vi "纳清pH电极校准.vi"() -> ()   [LabVIEW 2016, in "斯坦道多参数.lvlib"]
uses:
  <vilib>/Utility/miscctls.llb/LVPointTypeDef.ctl
  <vilib>/Analysis/NI_AALBase.lvlib
panel:
  out "第二点信号值":dbl
  out "第一点信号值":dbl
  out "报警信息":string
  out "通讯状态":string
  out "第二点校准值":dbl
  out "第一点校准值":dbl
  in  "校准停止":bool
  in  "校准启动":bool
  in  "校准模式":enum16{"两点校准", "单点校准"}(ring)
  out "最小值":sgl format="%#.2f"
  out "最大值":sgl format="%#.2f"
  out "波形图表":dbl(graph) caption="历史曲线"
  out "mean":dbl caption="均值" format="%#.2f"
  out "standard deviation":dbl caption="标准差" format="%#.2f"
  out "变异系数":dbl format="%#.6f"
  out "测量值":sgl format="%#.2f"
  out "提示":string
  out "标液2":sgl
  out "标液1":sgl
  out "原始光强数值":sgl caption="信号值" format="%#.6f"
  out "温度":dbl format="%#.2f"
  # "pH电极设定"
  # "℃"
  # "mV"
  # "请选择校准模式:"
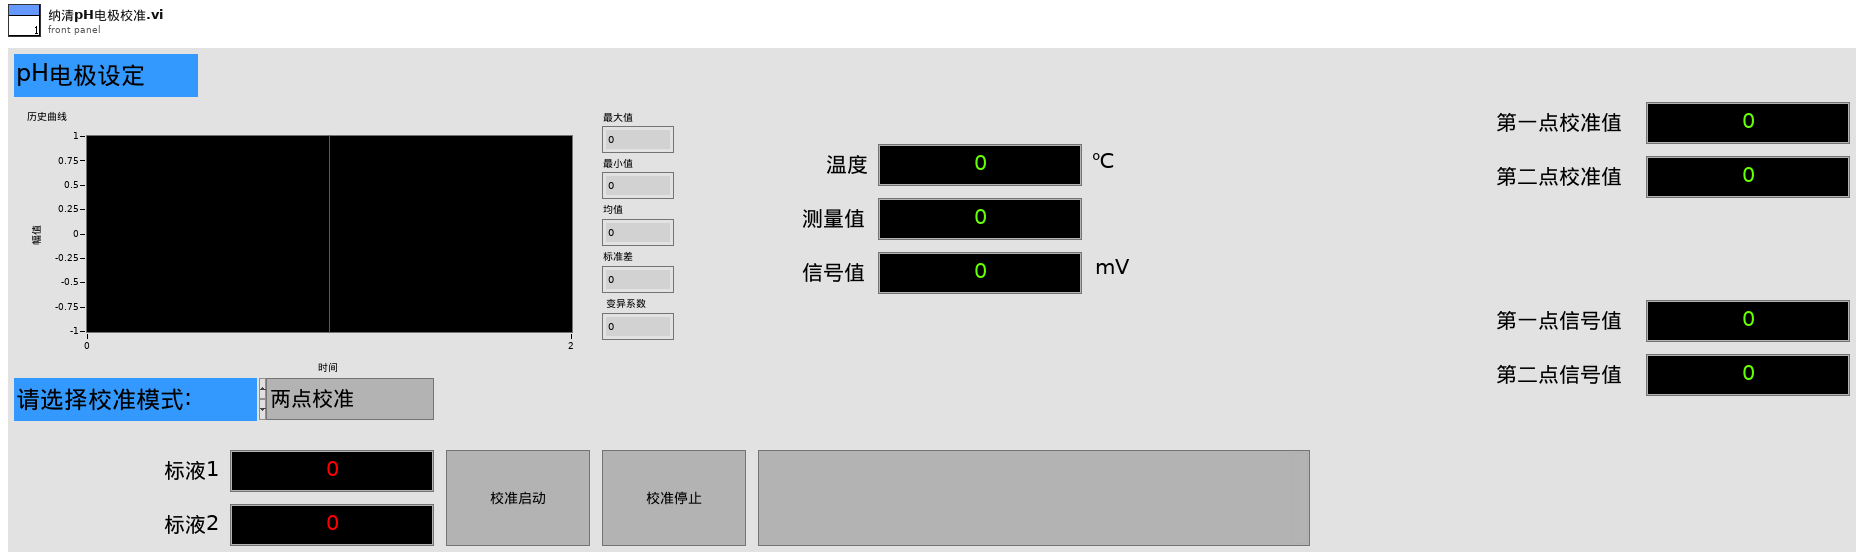
[diagram p1: front panel]
types:
  T1 = typedef "LVPointTypeDef.ctl" = cluster{"Horizontal":i16, "Vertical":i16}
  T2 = cluster{"报警码":u16, "pH数值":sgl, "0X0003_NC":sgl, "温度数据":sgl, "pH原始信号 mv":sgl, "0X0009_NC":string, "产品名称":string, "序列号":string, "硬件版本":string, "软件版本":string, "通讯地址":u16, "波特率":u16, "设备类型":u16, "0X0026_NC":string, "第一点原始数据":sgl, "第一点校准数据":sgl, "第二点原始数据":sgl, "第二点校准数据":sgl, "探头校准命令":u16, "温度校准参数":sgl, "温度校准命令":u16}
  T3 = enum8{"Enabled", "Disabled", "Disabled and Grayed Out"}
  T4 = cluster{"ph":bool, "DO":bool, "Cond":bool, "Turb":bool, "叶绿素a":bool, "藻密度":bool, "ORP":bool}
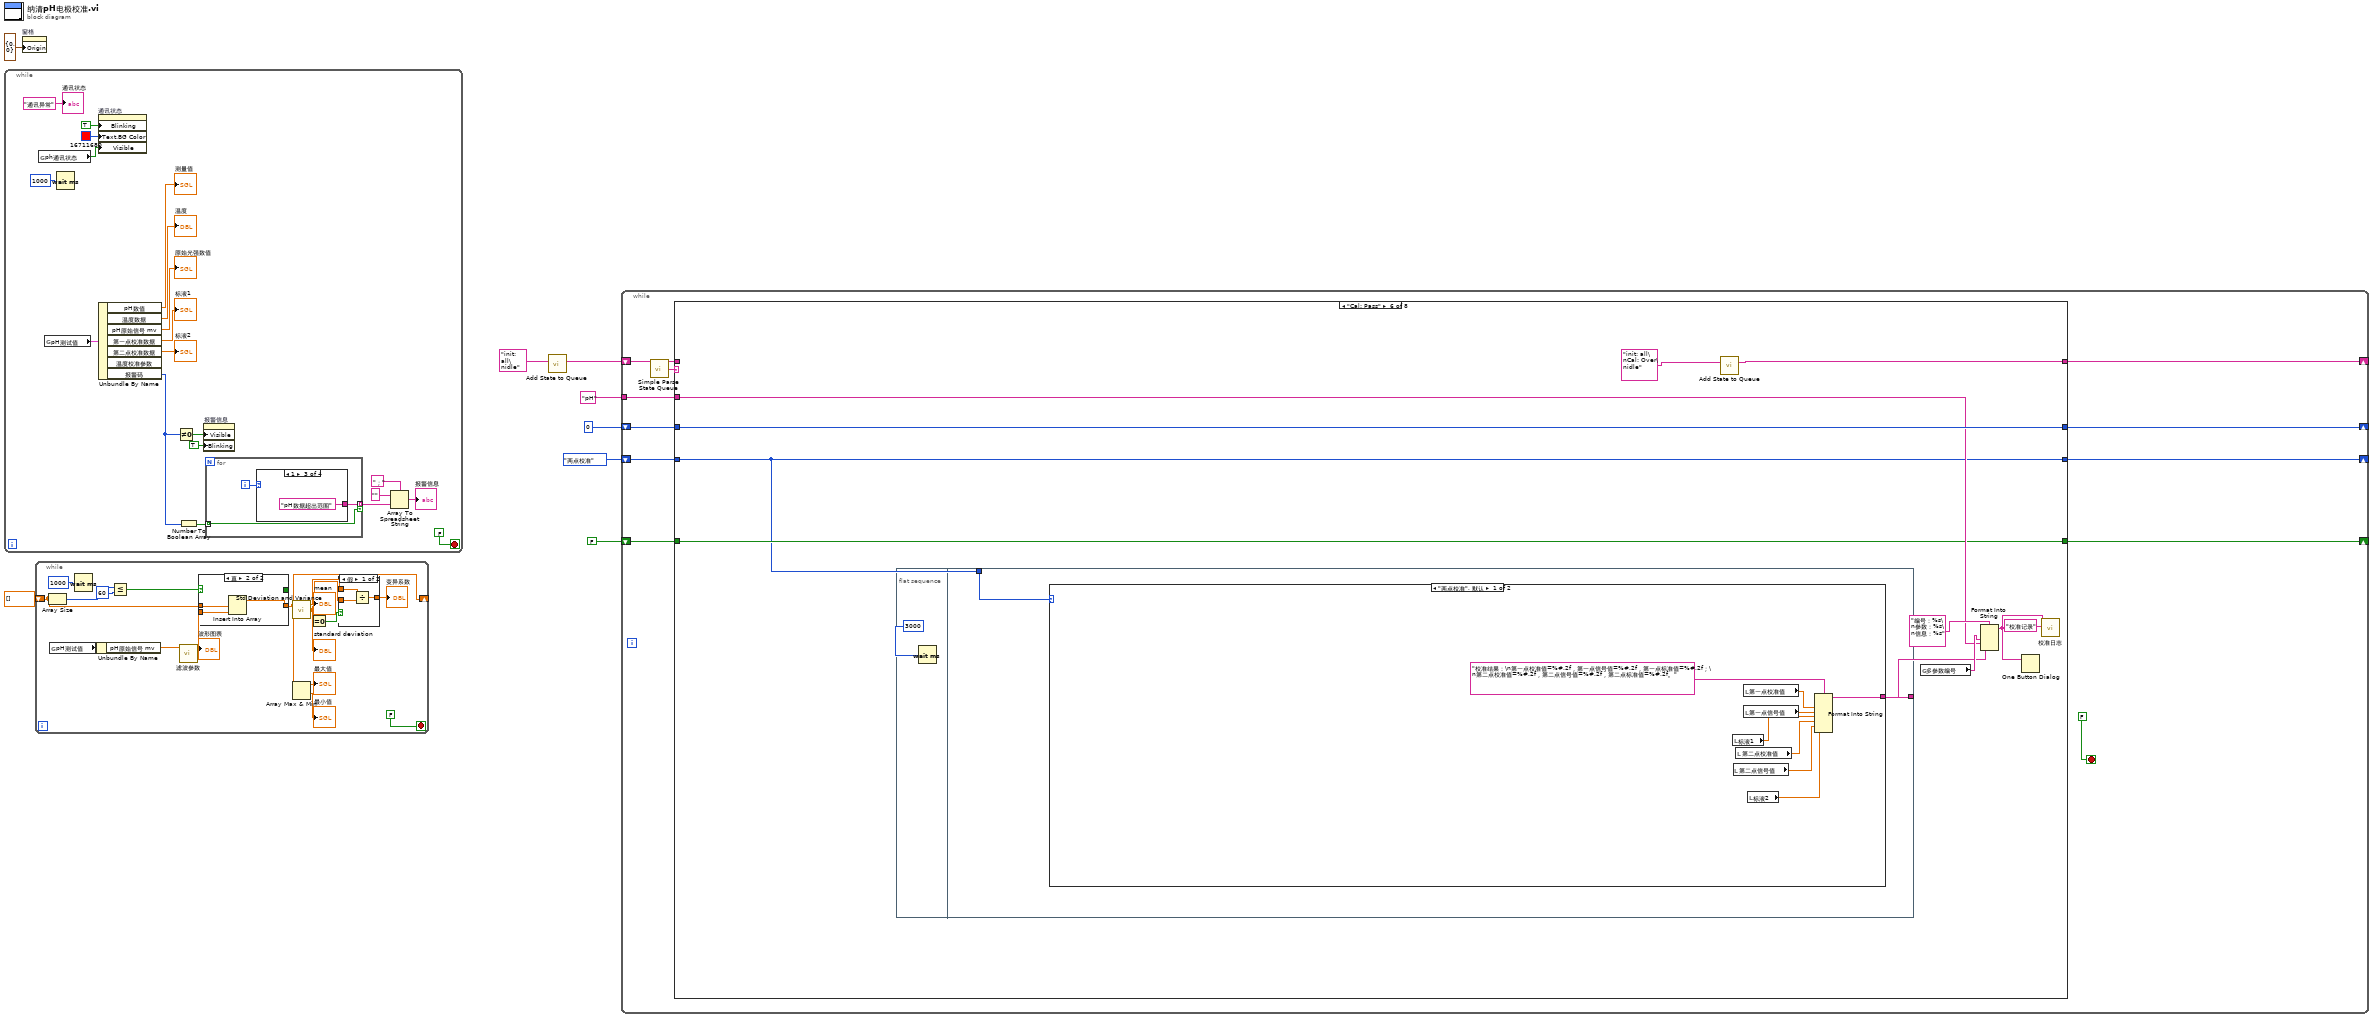
[diagram p0: block diagram]
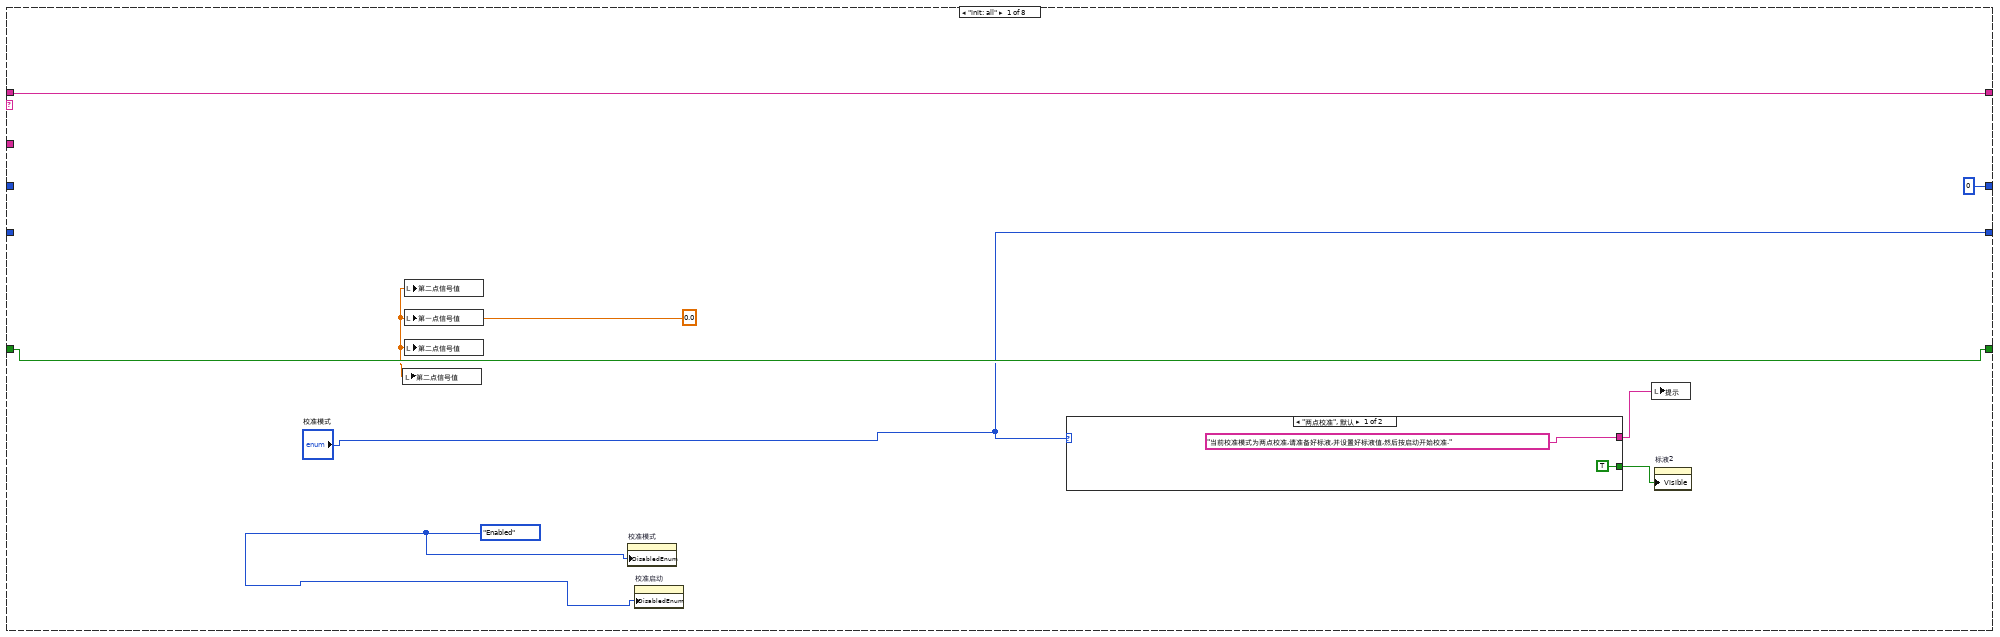
[diagram p2: hidden frame]
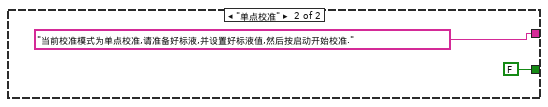
[diagram p3: hidden frame]
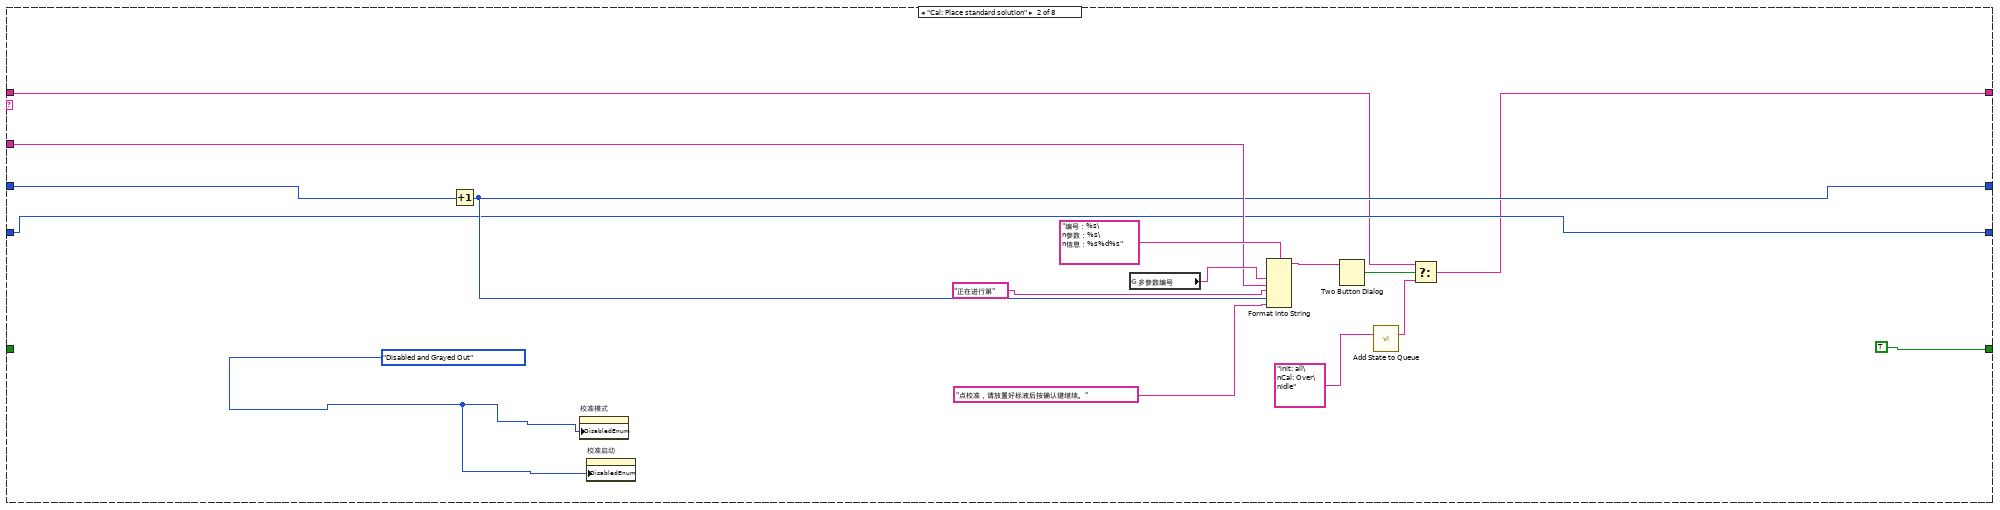
[diagram p4: hidden frame]
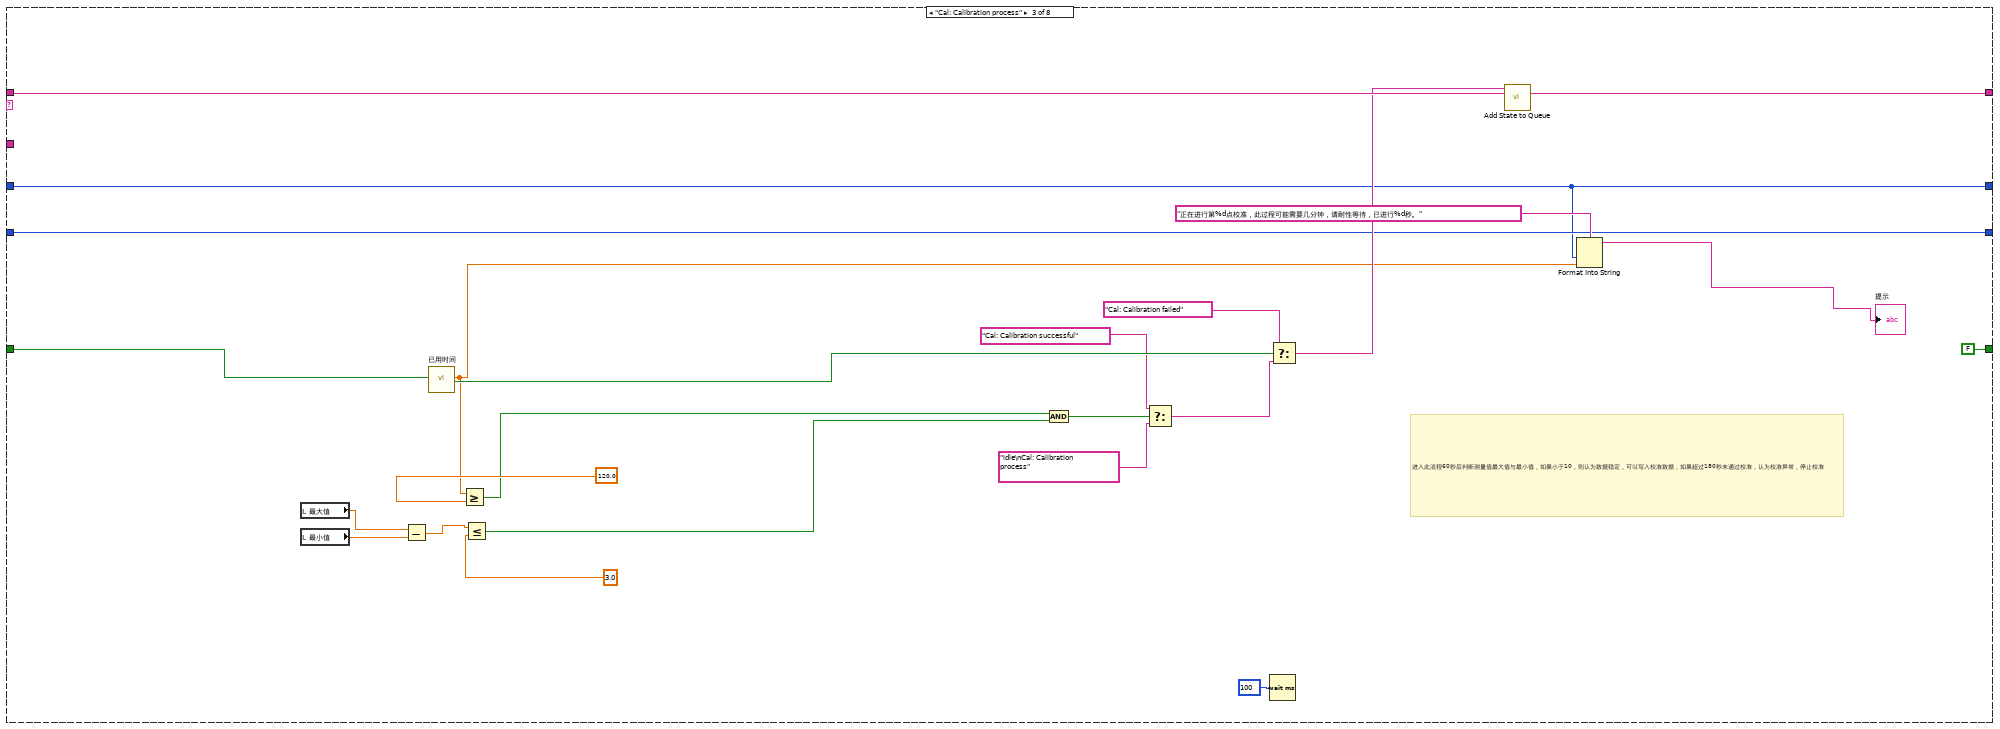
[diagram p5: hidden frame]
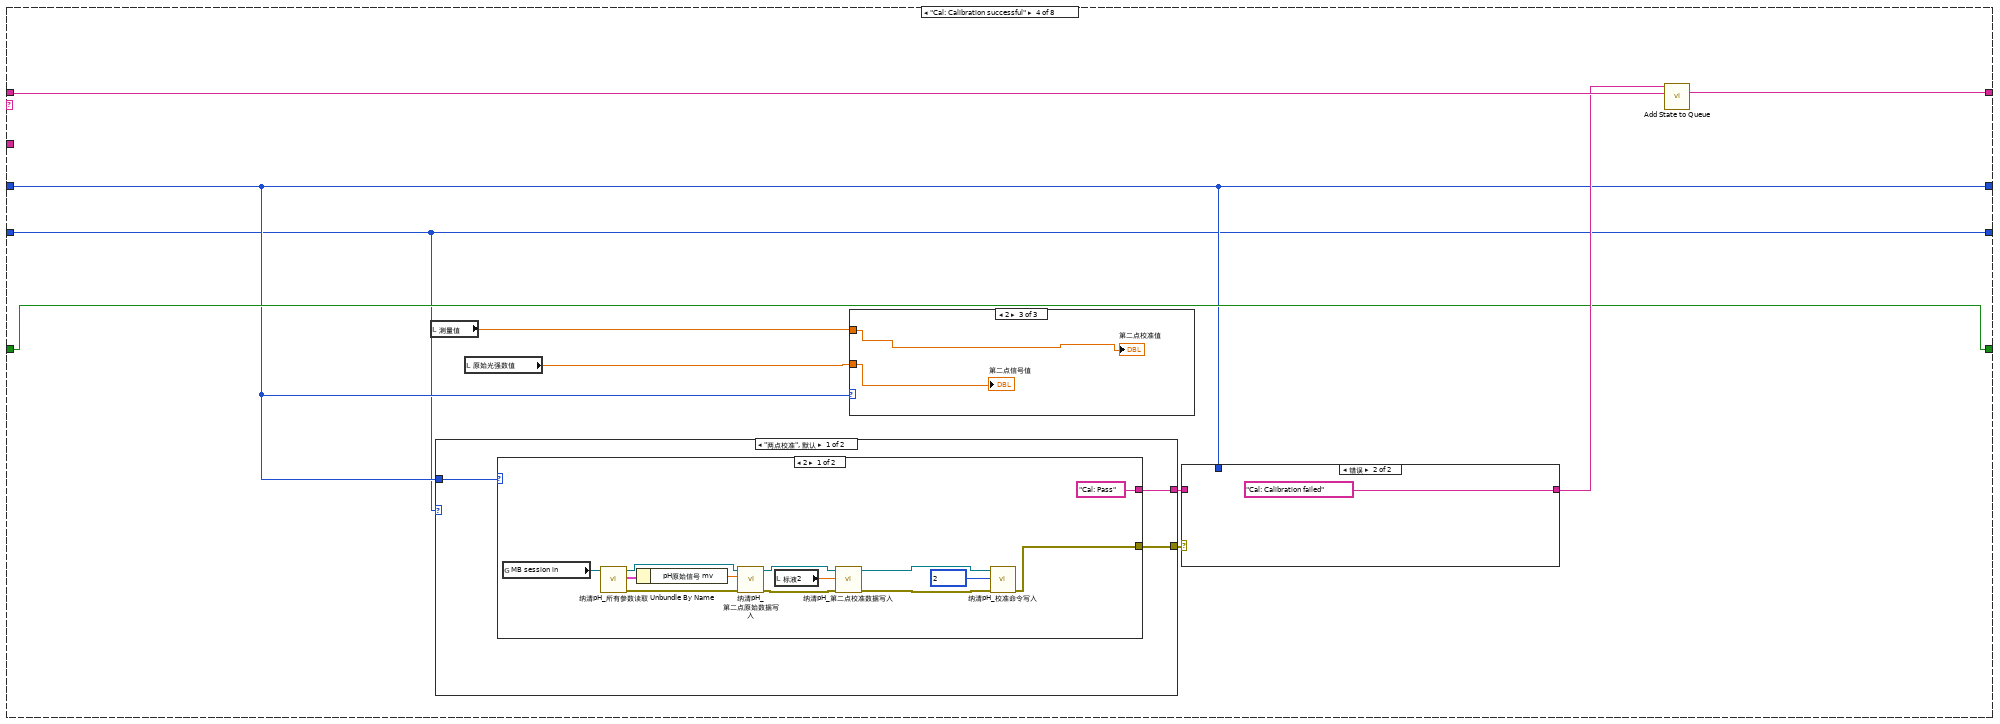
[diagram p6: hidden frame]
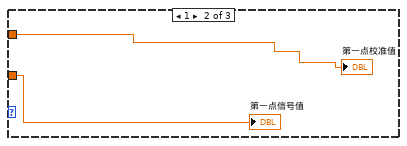
[diagram p8: hidden frame]
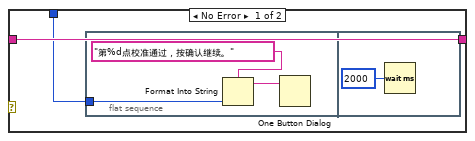
[diagram p9: hidden frame]
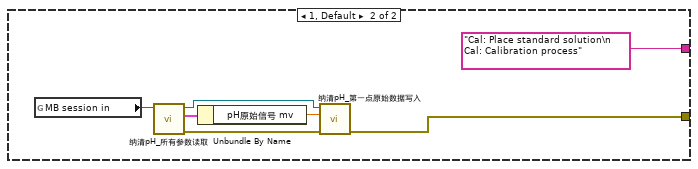
[diagram p10: hidden frame]
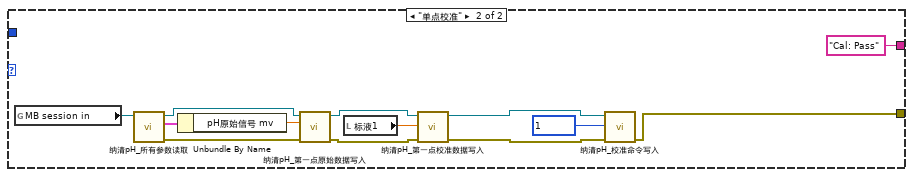
[diagram p11: hidden frame]
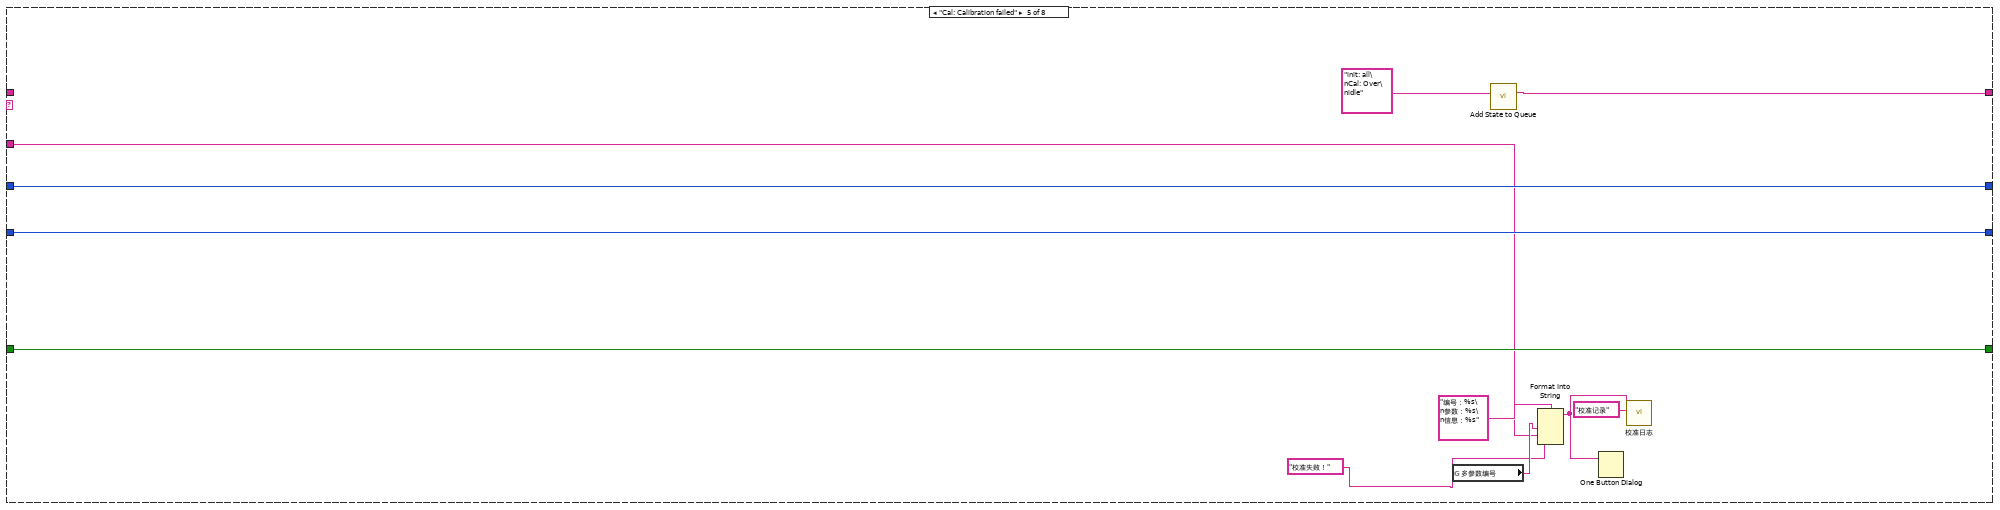
[diagram p12: hidden frame]
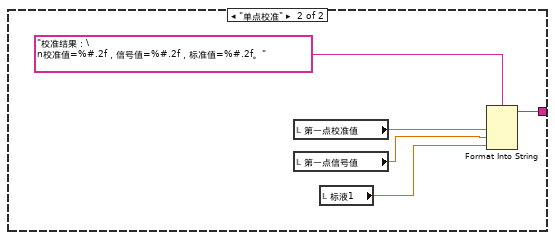
[diagram p13: hidden frame]
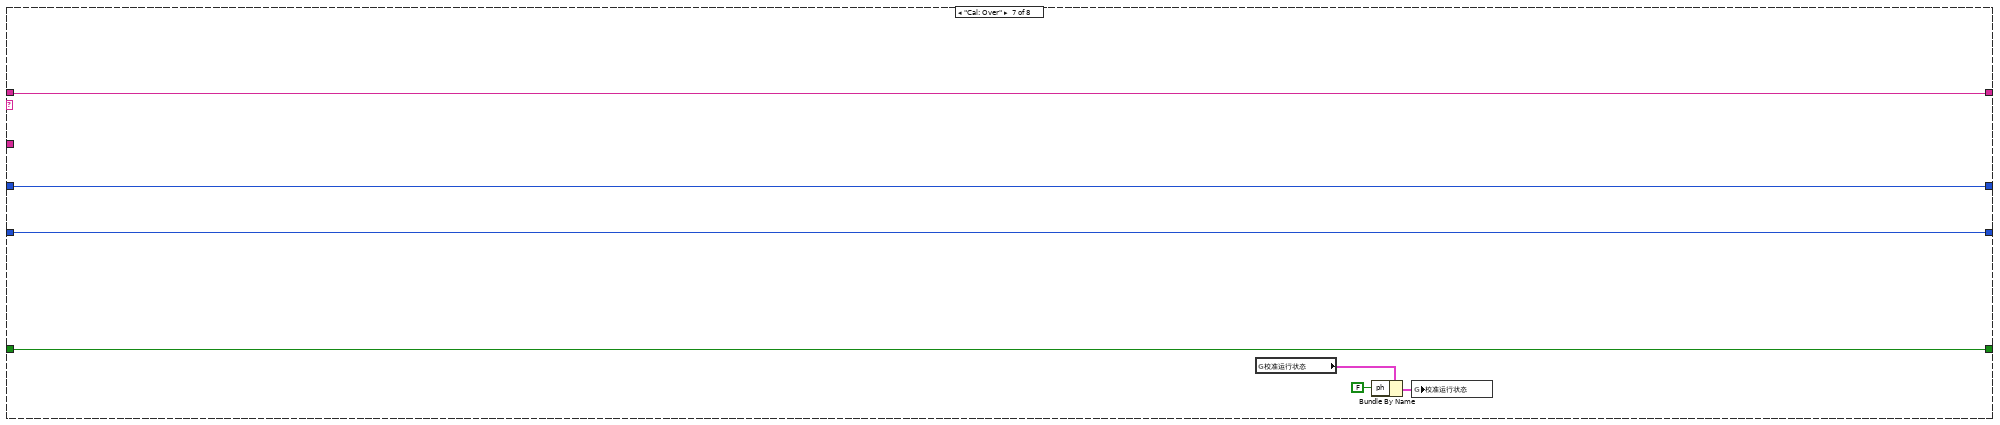
[diagram p14: hidden frame]
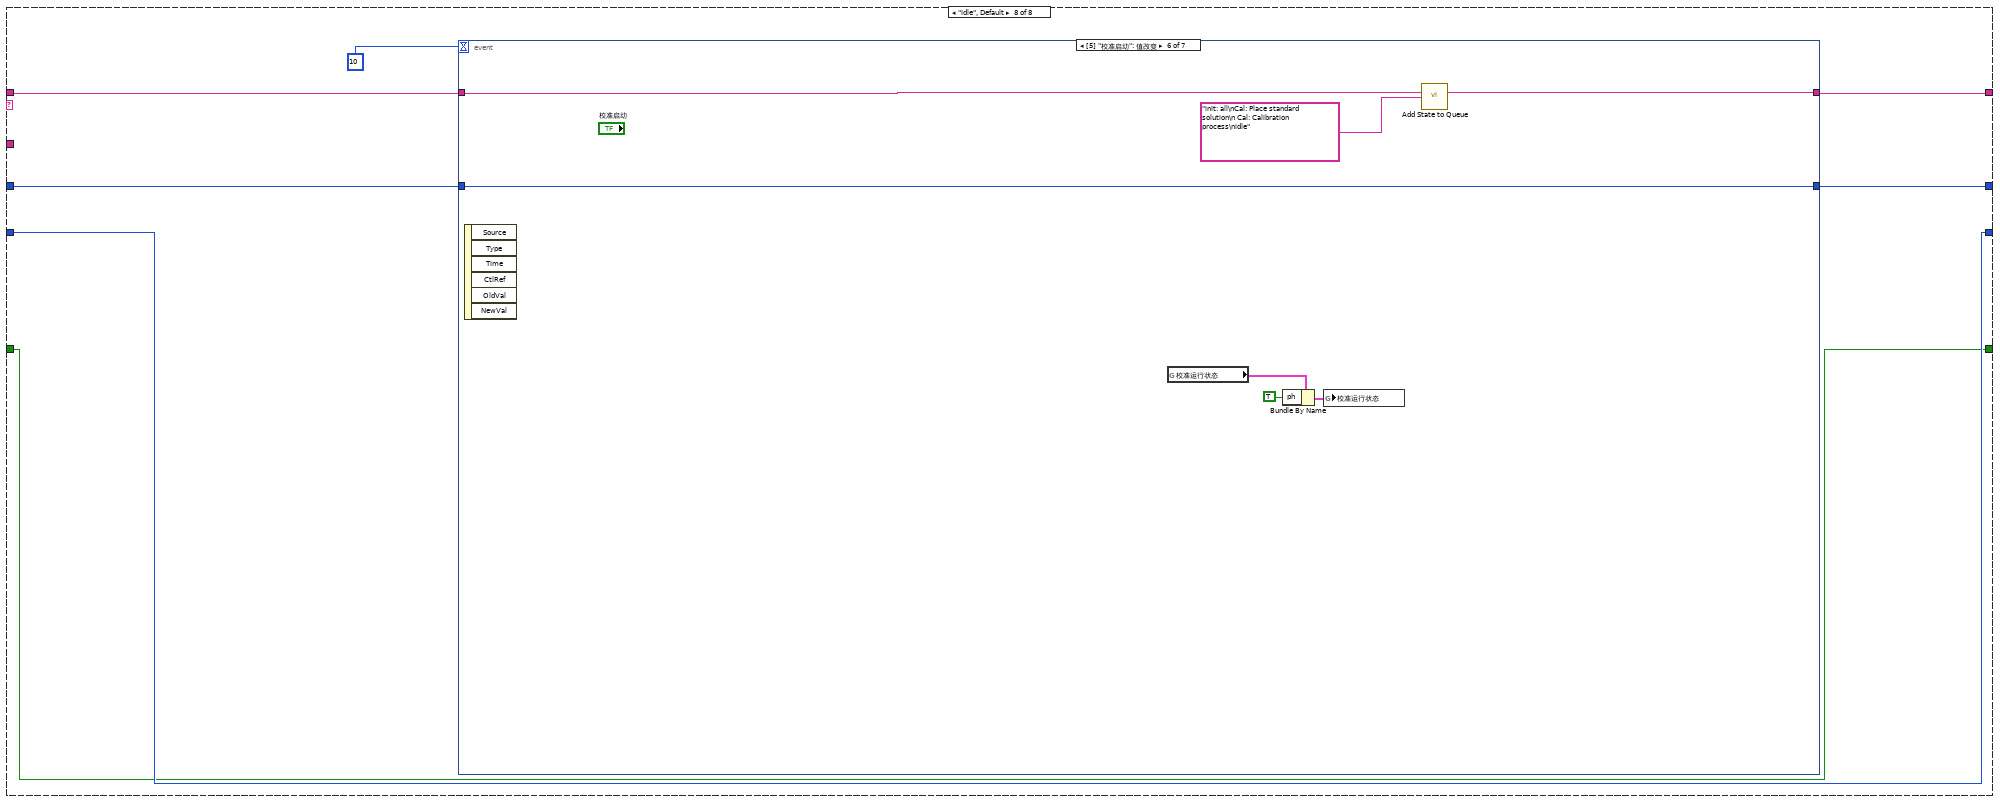
[diagram p15: hidden frame]
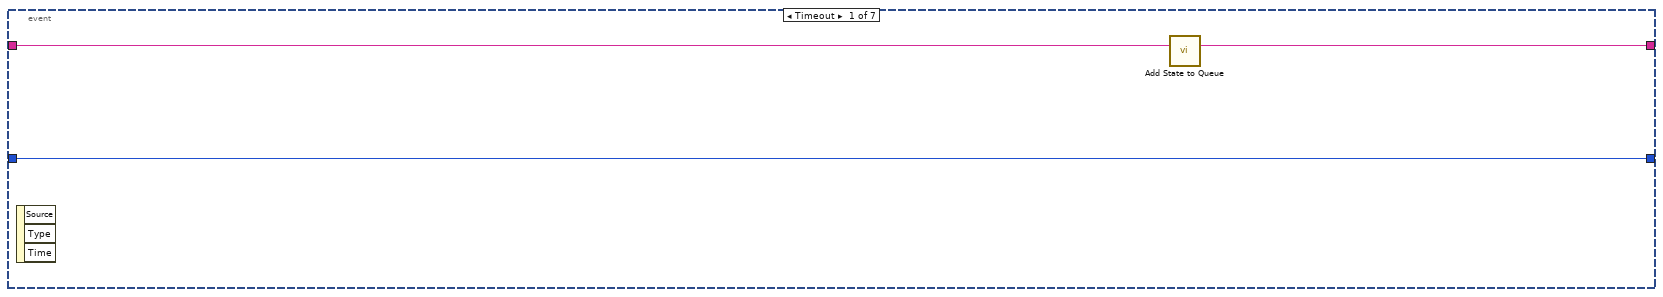
[diagram p16: hidden frame]
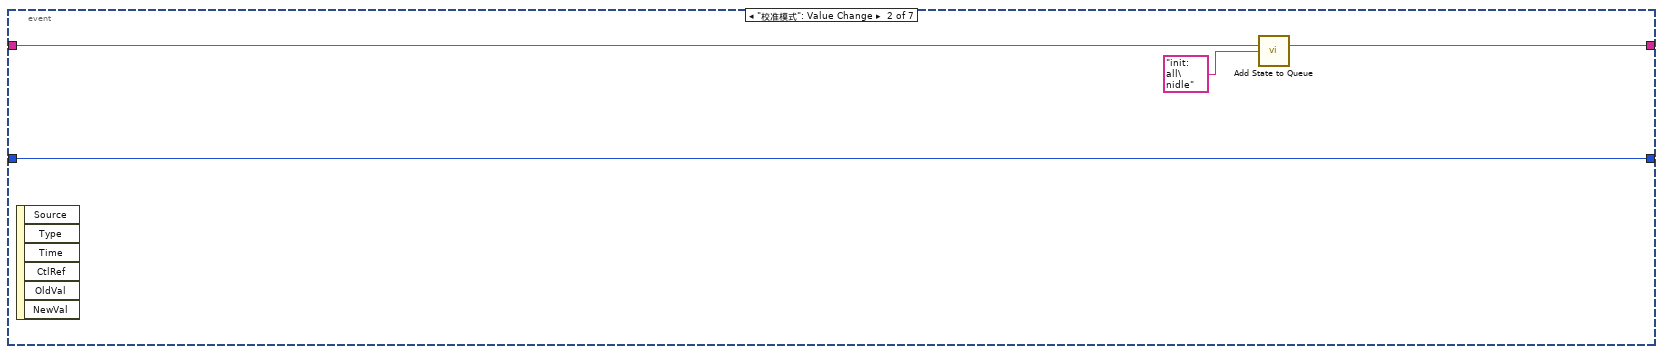
[diagram p17: hidden frame]
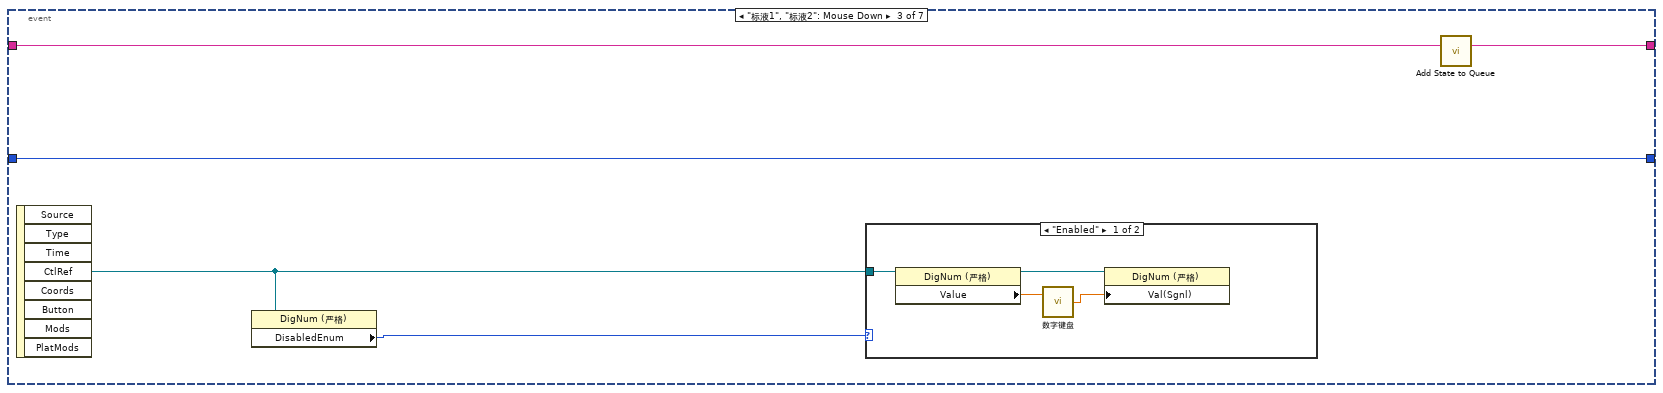
[diagram p18: hidden frame]
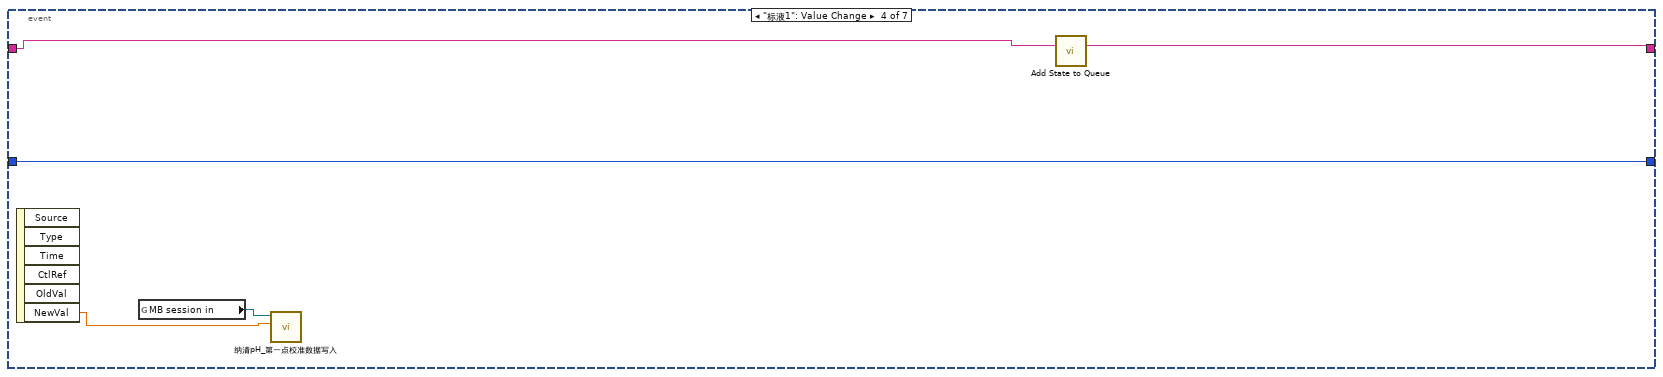
[diagram p20: hidden frame]
diagram:
  n1 = while {
    stop <- FALSE stop-if-true
    n2 = global read "多参数全局变量.vi" "ph通讯状态"() -> (w17:bool)
    n3 = global read "纳清过程全局变量.vi" "pH测试值"() -> (w26:T2)
    n4 = Wait (ms)(milliseconds to wait=u32 1000 ("等待时间（毫秒）")) -> ()  [unwired: 1 out]
    n5 = property on="通讯状态" class="Str"("Blinking"=TRUE ("闪烁"), "Text.BG Color"=u32 16711680, "Visible"=w17) -> ()  [unwired: 2 in, 2 out]
    n6 = Unbundle By Name(w26) -> ("pH数值"=→"测量值":sgl, "温度数据"=→"温度":sgl, "pH原始信号 mv"=→"原始光强数值":sgl, "第一点校准数据"=→"标液1":sgl, "第二点校准数据"=→"标液2":sgl, "报警码"=w11:u16)  [unwired: 1 out]
    n7 = Not Equal To 0?(x=w11) -> (x != 0?=w10:bool)
    n8 = Number To Boolean Array(number=w11) -> (Boolean array=w16:bool[])
    n9 = property on="报警信息" class="Str"("Visible"=w10, "Blinking"=TRUE ("闪烁")) -> ()  [unwired: 2 in, 2 out]
    n10 = for {
      tunnel: w16 -> [w29] mode=indexing
      tunnel: [w30] -> w15 mode=indexing if=w29
      i -> [w31]
      n11 = case shown="1" w31 {
        tunnel: [_ "温度超出范围" "pH数据超出范围" "温度传感器故障"] -> w30
        frame Default {
        }
        frame 0 {
        }
        frame 1 {
        }
        frame 8 {
        }
      }
    }
    n12 = Array To Spreadsheet String(delimiter (Tab)="；" ("分隔符(Tab)"), array=w15, 3:"" ("格式字符串")) -> (spreadsheet string=→"报警信息":string)
    "通讯状态" <- "通讯异常" ("当前串口")
  }
  n13 = property on="窗格" class="Pane"("Origin"=T1 {"Horizontal"=0, "Vertical"=0} ("原点")) -> ()  [unwired: 2 in, 2 out]
  n14 = while {
    shift-right: [w40] -> _
    shift-left: sgl[] [] -> [w46]
    stop <- FALSE stop-if-true
    n15 = Array Size(array=w46) -> (size(s)=w48:i32)
    n16 = global read "纳清过程全局变量.vi" "pH测试值"() -> (w37:T2)
    n17 = Wait (ms)(milliseconds to wait=u32 1000 ("等待时间（毫秒）")) -> ()  [unwired: 1 out]
    n18 = Unbundle By Name(w37) -> ("pH原始信号 mv"=w36:sgl)
    n19 = Less Or Equal?(x=w48, y=60) -> (x <= y?=w47:bool)
    n20 = call "滤波参数.vi"("x"=w36) -> ("mode"=w35:dbl)  [unwired: 10 in]
    "波形图表" <- w35
    n21 = case shown="真" w47 {
      tunnel: w46 -> [w59 w62]
      tunnel: w35 -> [w57 w61]
      tunnel: [w55 w60] -> w40
      tunnel: [TRUE _] -> _
      frame False {
        n22 = Replace Array Subset(array=w59, new element=w57) -> (w58:sgl[])  [unwired: 1 in]
        n23 = Rotate 1D Array(1:w58, 2:-1 ("n")) -> (0:w55:sgl[])
      }
      frame True {
        n24 = Insert Into Array(array=w62, new element=w61) -> (w60:sgl[])  [unwired: 1 in]
      }
    }
    n25 = call <vilib>:"Std Deviation and Variance.vi"("X"=w40) -> ("mean"=w44:dbl, "standard deviation"=w43:dbl)  [unwired: 1 in, 1 out]
    "mean" <- w44
    "standard deviation" <- w43
    n26 = Array Max & Min(array=w40) -> (max value=→"最大值":sgl, min value=→"最小值":sgl)  [unwired: 2 out]
    n27 = Equal To 0?(x=w44) -> (x = 0?=w45:bool)
    n28 = case shown="假" w45 {
      tunnel: w43 -> [w53 _]
      tunnel: [w52 _] -> w42
      tunnel: w44 -> [w51 _]
      frame False {
        n29 = Divide(x=w53, y=w51) -> (x/y=w52:dbl)
      }
      frame True {
      }
    }
    "变异系数" <- w42
  }
  n30 = call "Add State to Queue.vi"("State(s) In (\"\")"="init: all\nidle" ("State(s) In (\"\")")) -> ("States Out"=w5:string)  [unwired: 14 in]
  n31 = while {
    shift-right: [w70] -> _
    shift-left: w5 -> [w74]
    shift-right: [w67] -> _
    shift-left: 0 -> [w69]
    tunnel: "pH" ("State(s) In (\"\")") -> [w68]
    shift-right: [w65] -> _
    shift-left: enum16{"两点校准", "单点校准"}."两点校准" ("校准模式") -> [w66]
    shift-right: [w63] -> _
    shift-left: FALSE -> [w64]
    stop <- FALSE stop-if-true
    n32 = call "Simple Parse State Queue.vi"("State Queue"=w74) -> ("Remain States"=w71:string, "Next State"=w72:string)  [unwired: 13 in]
    n33 = case shown="\"Cal: Pass\"" w72 {
      tunnel: w71 -> [w82 w90 w121 w134 _ _ w228 w235]
      tunnel: [w82 w89 w120 w133 w191 w196 w228 w234] -> w70
      tunnel: w69 -> [_ w98 w105 w128 w194 w205 w227 w232]
      tunnel: w68 -> [_ w99 _ _ w185 w201 _ _]
      tunnel: [0 w96 w105 w128 w194 w205 w227 w233] -> w67
      tunnel: w66 -> [_ w95 w106 w127 w193 w197 w226 w231]
      tunnel: ["校准模式" w95 w106 w127 w193 w197 w226 w231] -> w65
      tunnel: w64 -> [w79 _ w108 w129 w192 w200 w225 w229]
      tunnel: [w79 TRUE FALSE w129 w192 w200 w225 w229] -> w63
      frame "init: all" {
        w77 = T3."Enabled" ("禁用")
        w78 = 0.0 ("第一点校准值")
        n34 = local write "第二点信号值"(w78) -> ()
        n35 = local write "第二点信号值"(w78) -> ()
        n36 = local write "第一点信号值"(w78) -> ()
        n37 = local write "第二点信号值"(w78) -> ()
        n38 = property on="校准模式" class="Enum (严格)"("DisabledEnum"=w77) -> ()  [unwired: 2 in, 2 out]
        n39 = property on="校准启动" class="Bool"("DisabledEnum"=w77) -> ()  [unwired: 2 in, 2 out]
        n40 = case shown="\"两点校准\", 默认" "校准模式" {
          tunnel: ["当前校准模式为两点校准,请准备好标液,并设置好标液值,然后按启动开始校准." ("提示") "当前校准模式为单点校准,请准备好标液,并设置好标液值,然后按启动开始校准." ("提示")] -> w81
          tunnel: [TRUE ("可见") FALSE ("可见")] -> w75
          frame "两点校准", Default {
          }
          frame "单点校准" {
          }
        }
        n41 = local write "提示"(w81) -> ()
        n42 = property on="标液2" class="DigNum (严格)"("Visible"=w75) -> ()  [unwired: 2 in, 2 out]
      }
      frame "Cal: Place standard solution" {
        w88 = T3."Disabled and Grayed Out" ("禁用")
        n43 = Increment(x=w98) -> (x+1=w96:i32)
        n44 = property on="校准模式" class="Enum (严格)"("DisabledEnum"=w88) -> ()  [unwired: 2 in, 2 out]
        n45 = property on="校准启动" class="Bool"("DisabledEnum"=w88) -> ()  [unwired: 2 in, 2 out]
        n46 = global read "多参数全局变量.vi" "多参数编号"() -> (w101:string)
        n47 = Format Into String(format string="编号：%s\n参数：%s\n信息：%s%d%s" ("格式字符串"), w101, w99, "正在进行第" ("消息"), w96, "点校准，请放置好标液后按确认键继续。" ("消息")) -> (resulting string=w93:string)  [unwired: 2 in, 1 out]
        n48 = Two Button Dialog(message=w93) -> (T button?=w92:bool)  [unwired: 2 in]
        n49 = call "Add State to Queue.vi"("State(s) In (\"\")"="init: all\nCal: Over\nidle" ("State(s) In (\"\")")) -> ("States Out"=w91:string)  [unwired: 14 in]
        n50 = Select(t=w90, s=w92, f=w91) -> (s? t:f=w89:string)
      }
      frame "Cal: Calibration process" {
        # "进入此流程60秒后判断测量值最大值与最小值，如果小于10，则认为数据稳定，可以写入校准数据，如果超过180秒未通过校准，认为校准异常，停止校准"
        n51 = local read "最大值"() -> (w125:sgl)
        n52 = local read "最小值"() -> (w124:sgl)
        n53 = Subtract(x=w125, y=w124) -> (x-y=w126:sgl)
        n54 = call "已用时间"("Reset"=w108) -> ("Elapsed Time (s)"=w104:dbl, "Time has Elapsed"=w122:bool)  [unwired: 11 in, 6 out]
        n55 = Greater Or Equal?(x=w104, y=120.0) -> (x >= y?=w117:bool)
        n56 = Less Or Equal?(x=w126, y=3.0) -> (x <= y?=w113:bool)
        n57 = And(x=w117, y=w113) -> (x .and. y?=w114:bool)
        n58 = Select(t="Cal: Calibration successful" ("State(s) In (\"\")"), s=w114, f="idle\nCal: Calibration process" ("State(s) In (\"\")")) -> (s? t:f=w112:string)
        n59 = Wait (ms)(milliseconds to wait=u32 100 ("等待时间（毫秒）")) -> ()  [unwired: 1 out]
        n60 = Select(t="Cal: Calibration failed" ("State(s) In (\"\")"), s=w122, f=w112) -> (s? t:f=w111:string)
        n61 = call "Add State to Queue.vi"("State(s) In Front (\"\")"=w111, "State(s) In (\"\")"=w121) -> ("States Out"=w120:string)  [unwired: 13 in]
        n62 = Format Into String(format string="正在进行第%d点校准，此过程可能需要几分钟，请耐性等待，已进行%d秒。" ("格式字符串"), w105, w104) -> (resulting string=→"提示":string)  [unwired: 2 in, 1 out]
      }
      frame "Cal: Calibration successful" {
        n63 = local read "测量值"() -> (w130:sgl)
        n64 = case shown="\"两点校准\", 默认" w127 {
          tunnel: [w150 w171] -> w136
          tunnel: [w149 "Cal: Pass" ("State(s) In (\"\")")] -> w135
          tunnel: w128 -> [w148 _]
          frame "两点校准", Default {
            n65 = case shown="2" w148 {
              tunnel: [w151 w164] -> w150
              tunnel: ["Cal: Pass" ("State(s) In (\"\")") "Cal: Place standard solution\n Cal: Calibration process" ("State(s) In (\"\")")] -> w149
              frame 2 {
                n66 = global read "多参数全局变量.vi" "MB session in"() -> (w159:refnum<class "MB_Master.lvclass">)
                n67 = call "纳清pH_所有参数读取.vi"("MB session in"=w159) -> ("error out"=w161:errorcluster, "输出值"=w158:T2, "MB session out"=w160:refnum<class "MB_Master.lvclass">)  [unwired: 8 in]
                n68 = Unbundle By Name(w158) -> ("pH原始信号 mv"=w157:sgl)
                n69 = call "纳清pH_第二点原始数据写入.vi"("error in (no error)"=w161, "数值"=w157, "MB session in"=w160) -> ("error out"=w156:errorcluster, "MB session out"=w155:refnum<class "MB_Master.lvclass">)  [unwired: 7 in]
                n70 = local read "标液2"() -> (w152:sgl)
                n71 = call "纳清pH_第二点校准数据写入.vi"("error in (no error)"=w156, "数值"=w152, "MB session in"=w155) -> ("error out"=w154:errorcluster, "MB session out"=w153:refnum<class "MB_Master.lvclass">)  [unwired: 7 in]
                n72 = call "纳清pH_校准命令写入.vi"("error in (no error)"=w154, "数值"=u16 2 ("starting address"), "MB session in"=w153) -> ("error out"=w151:errorcluster)  [unwired: 7 in, 1 out]
              }
              frame 1, Default {
                n73 = global read "多参数全局变量.vi" "MB session in"() -> (w167:refnum<class "MB_Master.lvclass">)
                n74 = call "纳清pH_所有参数读取.vi"("MB session in"=w167) -> ("error out"=w169:errorcluster, "输出值"=w166:T2, "MB session out"=w168:refnum<class "MB_Master.lvclass">)  [unwired: 8 in]
                n75 = Unbundle By Name(w166) -> ("pH原始信号 mv"=w165:sgl)
                n76 = call "纳清pH_第一点原始数据写入.vi"("error in (no error)"=w169, "数值"=w165, "MB session in"=w168) -> ("error out"=w164:errorcluster)  [unwired: 7 in, 1 out]
              }
            }
          }
          frame "单点校准" {
            n77 = global read "多参数全局变量.vi" "MB session in"() -> (w179:refnum<class "MB_Master.lvclass">)
            n78 = call "纳清pH_所有参数读取.vi"("MB session in"=w179) -> ("error out"=w181:errorcluster, "输出值"=w178:T2, "MB session out"=w180:refnum<class "MB_Master.lvclass">)  [unwired: 8 in]
            n79 = Unbundle By Name(w178) -> ("pH原始信号 mv"=w177:sgl)
            n80 = call "纳清pH_第一点原始数据写入.vi"("error in (no error)"=w181, "数值"=w177, "MB session in"=w180) -> ("error out"=w176:errorcluster, "MB session out"=w175:refnum<class "MB_Master.lvclass">)  [unwired: 7 in]
            n81 = local read "标液1"() -> (w172:sgl)
            n82 = call "纳清pH_第一点校准数据写入.vi"("error in (no error)"=w176, "数值"=w172, "MB session in"=w175) -> ("error out"=w174:errorcluster, "MB session out"=w173:refnum<class "MB_Master.lvclass">)  [unwired: 7 in]
            n83 = call "纳清pH_校准命令写入.vi"("error in (no error)"=w174, "数值"=u16 1 ("starting address"), "MB session in"=w173) -> ("error out"=w171:errorcluster)  [unwired: 7 in, 1 out]
          }
        }
        n84 = local read "原始光强数值"() -> (w131:sgl)
        n85 = case shown="2" w128 {
          tunnel: w131 -> [_ w138 w140]
          tunnel: w130 -> [_ w137 w139]
          frame 0, Default {
          }
          frame 1 {
            "第一点信号值" <- w138
            "第一点校准值" <- w137
          }
          frame 2 {
            "第二点信号值" <- w140
            "第二点校准值" <- w139
          }
        }
        n86 = case shown="错误" w136 {
          tunnel: w135 -> [w142 _]
          tunnel: [w142 "Cal: Calibration failed" ("State(s) In (\"\")")] -> w132
          tunnel: w128 -> [w141 _]
          frame No Error {
            n87 = flat-sequence {
              tunnel: w141 -> [w143]
              frame #0 {
                n88 = Format Into String(format string="第%d点校准通过，按确认继续。" ("格式字符串"), w143) -> (resulting string=w145:string)  [unwired: 2 in, 1 out]
                n89 = One Button Dialog(message=w145) -> ()  [unwired: 1 in, 1 out]
              }
              frame #1 {
                n90 = Wait (ms)(milliseconds to wait=u32 2000 ("等待时间（毫秒）")) -> ()  [unwired: 1 out]
              }
            }
          }
          frame Error {
          }
        }
        n91 = call "Add State to Queue.vi"("State(s) In Front (\"\")"=w132, "State(s) In (\"\")"=w134) -> ("States Out"=w133:string)  [unwired: 13 in]
      }
      frame "Cal: Calibration failed" {
        n92 = global read "多参数全局变量.vi" "多参数编号"() -> (w188:string)
        n93 = call "Add State to Queue.vi"("State(s) In (\"\")"="init: all\nCal: Over\nidle" ("State(s) In (\"\")")) -> ("States Out"=w191:string)  [unwired: 14 in]
        n94 = Format Into String(format string="编号：%s\n参数：%s\n信息：%s" ("格式字符串"), w188, w185, "校准失败！" ("消息")) -> (resulting string=w187:string)  [unwired: 2 in, 1 out]
        n95 = One Button Dialog(message=w187) -> ()  [unwired: 1 in, 1 out]
        n96 = call "校准日志.vi"("table"="校准记录", "日志信息"=w187) -> ()  [unwired: 9 in, 1 out]
      }
      frame "Cal: Pass" {
        n97 = flat-sequence {
          tunnel: [w208] -> w198
          tunnel: w197 -> [w207]
          frame #0 {
            n98 = Wait (ms)(milliseconds to wait=u32 3000 ("等待时间（毫秒）")) -> ()  [unwired: 1 out]
          }
          frame #1 {
            n99 = case shown="\"两点校准\", 默认" w207 {
              tunnel: [w216 w221] -> w208
              frame "两点校准", Default {
                n100 = local read "标液1"() -> (w212:sgl)
                n101 = local read "第二点信号值"() -> (w210:dbl)
                n102 = local read "第二点校准值"() -> (w211:dbl)
                n103 = local read "第一点校准值"() -> (w214:dbl)
                n104 = local read "第一点信号值"() -> (w215:dbl)
                n105 = local read "标液2"() -> (w209:sgl)
                n106 = Format Into String(format string="校准结果：\n第一点校准值=%#.2f，第一点信号值=%#.2f，第一点标准值=%#.2f；\n第二点校准值=%#.2f，第二点信号值=%#.2f，第二点标准值=%#.2f。" ("提示"), w214, w215, w212, w211, w210, w209) -> (resulting string=w216:string)  [unwired: 2 in, 1 out]
              }
              frame "单点校准" {
                n107 = local read "第一点校准值"() -> (w220:dbl)
                n108 = local read "第一点信号值"() -> (w218:dbl)
                n109 = local read "标液1"() -> (w217:sgl)
                n110 = Format Into String(format string="校准结果：\n校准值=%#.2f，信号值=%#.2f，标准值=%#.2f。" ("提示"), w220, w218, w217) -> (resulting string=w221:string)  [unwired: 2 in, 1 out]
              }
            }
          }
        }
        n111 = call "Add State to Queue.vi"("State(s) In (\"\")"="init: all\nCal: Over\nidle" ("State(s) In (\"\")")) -> ("States Out"=w196:string)  [unwired: 14 in]
        n112 = global read "多参数全局变量.vi" "多参数编号"() -> (w202:string)
        n113 = Format Into String(format string="编号：%s\n参数：%s\n信息：%s" ("格式字符串"), w202, w201, w198) -> (resulting string=w199:string)  [unwired: 2 in, 1 out]
        n114 = One Button Dialog(message=w199) -> ()  [unwired: 1 in, 1 out]
        n115 = call "校准日志.vi"("table"="校准记录", "日志信息"=w199) -> ()  [unwired: 9 in, 1 out]
      }
      frame "Cal: Over" {
        n116 = global read "多参数全局变量.vi" "校准运行状态"() -> (w223:T4)
        n117 = Bundle By Name(cluster=w223, "ph"=FALSE) -> (w224:T4)
        n118 = global write "多参数全局变量.vi" "校准运行状态"(w224) -> ()
      }
      frame "idle", Default {
        n119 = event shown="[5] \"校准启动\": 值改变" {
          selector: _ -> [_ _ _ _ _ _ _]
          dyn-events: _ -> [_ _ _ _ _ _ _]
          timeout: 10 -> [_ _ _ _ _ _ _]
          tunnel: w235 -> [w238 w242 w245 w252 w257 w268 _]
          tunnel: [w237 w241 w246 w256 w261 w267 w270] -> w234
          tunnel: [w236 w239 w247 w255 w260 w265 w271] -> w233
          tunnel: w232 -> [w236 w239 w247 w255 w260 w265 w271]
          event Timeout {
            n120 = event-data() -> ()  [unwired: 1 in, 3 out]
            n121 = call "Add State to Queue.vi"("State(s) In (\"\")"=w238) -> ("States Out"=w237:string)  [unwired: 14 in]
          }
          event "校准模式": Value Change {
            n122 = event-data() -> ()  [unwired: 1 in, 6 out]
            n123 = call "Add State to Queue.vi"("State(s) In (\"\")"=w242, "State(s) At Back (\"\")"="init: all\nidle" ("State(s) In (\"\")")) -> ("States Out"=w241:string)  [unwired: 13 in]
          }
          event "标液1", "标液2": Mouse Down {
            n124 = event-data() -> ("CtlRef"=w244:refnum<vi>)  [unwired: 1 in, 7 out]
            n125 = property class="DigNum (严格)"(reference=w244) -> ("DisabledEnum"=w243:T3)  [unwired: 1 in, 2 out]
            n126 = case shown="\"Enabled\"" w243 {
              tunnel: w244 -> [w251 _]
              frame "Enabled" {
                n127 = property class="DigNum (严格)"(reference=w251) -> (reference out=w248:refnum<vi>, "Value"=w249:sgl)  [unwired: 1 in, 1 out]
                n128 = call "数字键盘.vi"("OldNumber"=w249) -> ("NewNumber"=w250:dbl)  [unwired: 1 in]
                n129 = property class="DigNum (严格)"(reference=w248, "Val(Sgnl)"=w250) -> ()  [unwired: 1 in, 2 out]
              }
              frame "Disabled", Default {
              }
            }
            n130 = call "Add State to Queue.vi"("State(s) In (\"\")"=w245) -> ("States Out"=w246:string)  [unwired: 14 in]
          }
          event "标液1": Value Change {
            n131 = event-data() -> ("NewVal"=w253:sgl)  [unwired: 1 in, 5 out]
            n132 = global read "多参数全局变量.vi" "MB session in"() -> (w254:refnum<class "MB_Master.lvclass">)
            n133 = call "纳清pH_第一点校准数据写入.vi"("数值"=w253, "MB session in"=w254) -> ()  [unwired: 8 in, 2 out]
            n134 = call "Add State to Queue.vi"("State(s) In (\"\")"=w252) -> ("States Out"=w256:string)  [unwired: 14 in]
          }
          event "标液2": Value Change {
            n135 = event-data() -> ("NewVal"=w258:sgl)  [unwired: 1 in, 5 out]
            n136 = global read "多参数全局变量.vi" "MB session in"() -> (w259:refnum<class "MB_Master.lvclass">)
            n137 = call "纳清pH_第二点校准数据写入.vi"("数值"=w258, "MB session in"=w259) -> ()  [unwired: 8 in, 2 out]
            n138 = call "Add State to Queue.vi"("State(s) In (\"\")"=w257) -> ("States Out"=w261:string)  [unwired: 14 in]
          }
          event "校准启动": Value Change {
            n139 = event-data() -> ()  [unwired: 1 in, 6 out]
            n140 = global read "多参数全局变量.vi" "校准运行状态"() -> (w263:T4)
            n141 = Bundle By Name(cluster=w263, "ph"=TRUE) -> (w264:T4)
            n142 = global write "多参数全局变量.vi" "校准运行状态"(w264) -> ()
            n143 = call "Add State to Queue.vi"("State(s) In (\"\")"=w268, "State(s) At Back (\"\")"="init: all\nCal: Place standard solution\n Cal: Calibration process\nidle" ("State(s) In (\"\")")) -> ("States Out"=w267:string)  [unwired: 13 in]
          }
          event "校准停止": Value Change {
            n144 = event-data() -> ()  [unwired: 1 in, 6 out]
            n145 = call "Add State to Queue.vi"("State(s) In (\"\")"="init: all\nCal: Over\nidle" ("State(s) In (\"\")")) -> ("States Out"=w270:string)  [unwired: 14 in]
          }
        }
      }
    }
  }
